vi "rqcBob Mod Level Test - 2 SPD (Low Level Example).vi"() -> ()   [LabVIEW 2018]
uses:
  FPGA/rqcBob/Custom Controls/Pulse Train/rqcBob Pulse Train Config.ctl
  FPGA/rqcBob/Custom Controls/Pulse Train/rqcBob Pulse Train.Generation Mode.ctl
  FPGA/rqcBob/Custom Controls/Pulse Train/rqcBob Pulse Train.First Pulse Delay Mode.ctl
  FPGA/rqcBob/Custom Controls/rqcBob Modulator Config.ctl
  FPGA/rqcBob/Custom Controls/rqcBob Window Config.ctl
  Shared/Shared FPGA Lib/Shared Logic/Custom Controls/rqc Random Generator.parameters.ctl
  Shared/Shared FPGA Lib/Shared Logic/Custom Controls/rqc Random Generator.value type.ctl
  FPGA/rqcBob/Custom Controls/rqcBob Trigger Type.ctl
  <vilib>/Analysis/1siggen.llb/Ramp Pattern by Delta.vi
  <vilib>/FPGAPlugInAG/PCI-7811R/niLvFpga_Open_PCI-7811R.vi
  <vilib>/rvi/interface/common/dynamic/niFpgaDynamicAddResources.vi
  Low Level API/Configuration/Photon Detector/Detection FIFOs config/rqcBob Configure PD Detect FIFO (2PD).vi
  Low Level API/Read/Read PD Detection FIFO/rqcBob Read PD Detection FIFO (1PD PD1).vi
  Low Level API/Read/Read PD Detection FIFO/rqcBob Read PD Detection FIFO (1PD PD2).vi
  <vilib>/FPGAPlugInAG/Dynamic/niLvFpga_Close_Dynamic.vi
  <vilib>/rvi/interface/nirviOpenFPGA/nirviOpenFPGA.xnode
  FPGA Bitfiles/rqcBob (FPGA) 7811 v 4.0.0.lvbitx
  <vilib>/rvi/interface/nirviCloseFPGA/nirviCloseFPGA.xnode
  <vilib>/Analysis/NI_AALBase.lvlib
panel:
  out "Num of Detections (2-nd PD) vs DAC Level":cluster{u16[], "appended array":dbl[]}(graph)={[0, 8, 16, 24, 32, 40, 48, 56, 64, 72, 80, 88, 96, 104, 112, 120, 128, 136, 144, 152, 160, 168, 176, 184, 192, 200, 208, 216, 224, 232, 240, 248, 256, 264, 272, 280, 288, 296, 304, 312, 320, 328, 336, 344, 352, 360, 368, 376, 384, 392, 400, 408, 416, 424, 432, 440, 448, 456, 464, 472, 480, 488, 496, 504, 512], "appended array"=[0.0, 0.0, 0.0, 0.0, 0.0, 0.0, 0.0, 0.0, 0.0, 0.0, 0.0, 0.0, 0.0, 0.0, 0.0, 0.0, 0.0, 0.0, 0.0, 0.0, 0.0, 0.0, 0.0, 0.0, 0.0, 0.0, 0.0, 0.0, 0.0, 0.0, 0.0, 0.0, 0.0, 0.0, 0.0, 0.0, 0.0, 0.0, 0.0, 0.0, 0.0, 0.0, 0.0, 0.0, 0.0, 0.0, 0.0, 0.0, 0.0, 0.0, 0.0, 0.0, 0.0, 0.0, 0.0, 0.0, 0.0, 0.0, 0.0, 0.0, 0.0, 0.0, 0.0, 0.0, 0.0]}
  in  "modulator.clock delay":fxp<+,4,4> caption="PM Clock Delay (0-7) (in units of 40ns)"
  out "Progress":dbl(slide)=100.0 scale=0.0..100.0
  out "Num of Detections (1-st PD) vs DAC Level":cluster{u16[], "appended array":dbl[]}(graph)={[0, 8, 16, 24, 32, 40, 48, 56, 64, 72, 80, 88, 96, 104, 112, 120, 128, 136, 144, 152, 160, 168, 176, 184, 192, 200, 208, 216, 224, 232, 240, 248, 256, 264, 272, 280, 288, 296, 304, 312, 320, 328, 336, 344, 352, 360, 368, 376, 384, 392, 400, 408, 416, 424, 432, 440, 448, 456, 464, 472, 480, 488, 496, 504, 512], "appended array"=[0.0, 0.0, 0.0, 0.0, 0.0, 0.0, 0.0, 0.0, 0.0, 0.0, 0.0, 0.0, 0.0, 0.0, 0.0, 0.0, 0.0, 0.0, 0.0, 0.0, 0.0, 0.0, 0.0, 0.0, 0.0, 0.0, 0.0, 0.0, 0.0, 0.0, 0.0, 0.0, 0.0, 0.0, 0.0, 0.0, 0.0, 0.0, 0.0, 0.0, 0.0, 0.0, 0.0, 0.0, 0.0, 0.0, 0.0, 0.0, 0.0, 0.0, 0.0, 0.0, 0.0, 0.0, 0.0, 0.0, 0.0, 0.0, 0.0, 0.0, 0.0, 0.0, 0.0, 0.0, 0.0]}
  in  "stop":bool
  in  "DAC increment":u16=8
  in  "DAC Level max":u16=512
  in  "DAC Level min":u16
  in  "rndGen.parameters":T1={"value type"=enum."constant", "constant"=512, "num of levels"=0, "levels values"=[0, 0, 0, 0]} caption="Phase modulation value" {"num of levels" min=4 max=4 step=1}
  in  "window.config":T3 caption="Registration of detector clicks"
  in  "modulator.config":T4 caption="Phase modulation"
  in  "train.configuration":T5={"period"=0, "num of pulses"=0, "mode"=enum."train sequence.single", "num of trains"=0, "first pulse delay mode"=enum."every train", "first pulse delay"=55} caption="Pulsed laser configuration"
  out "Done":bool=TRUE
  # "PM Level Settings"
  # "Bob configuration"
  # "Advanced parameters"
  # "Constant"
  # "Random"
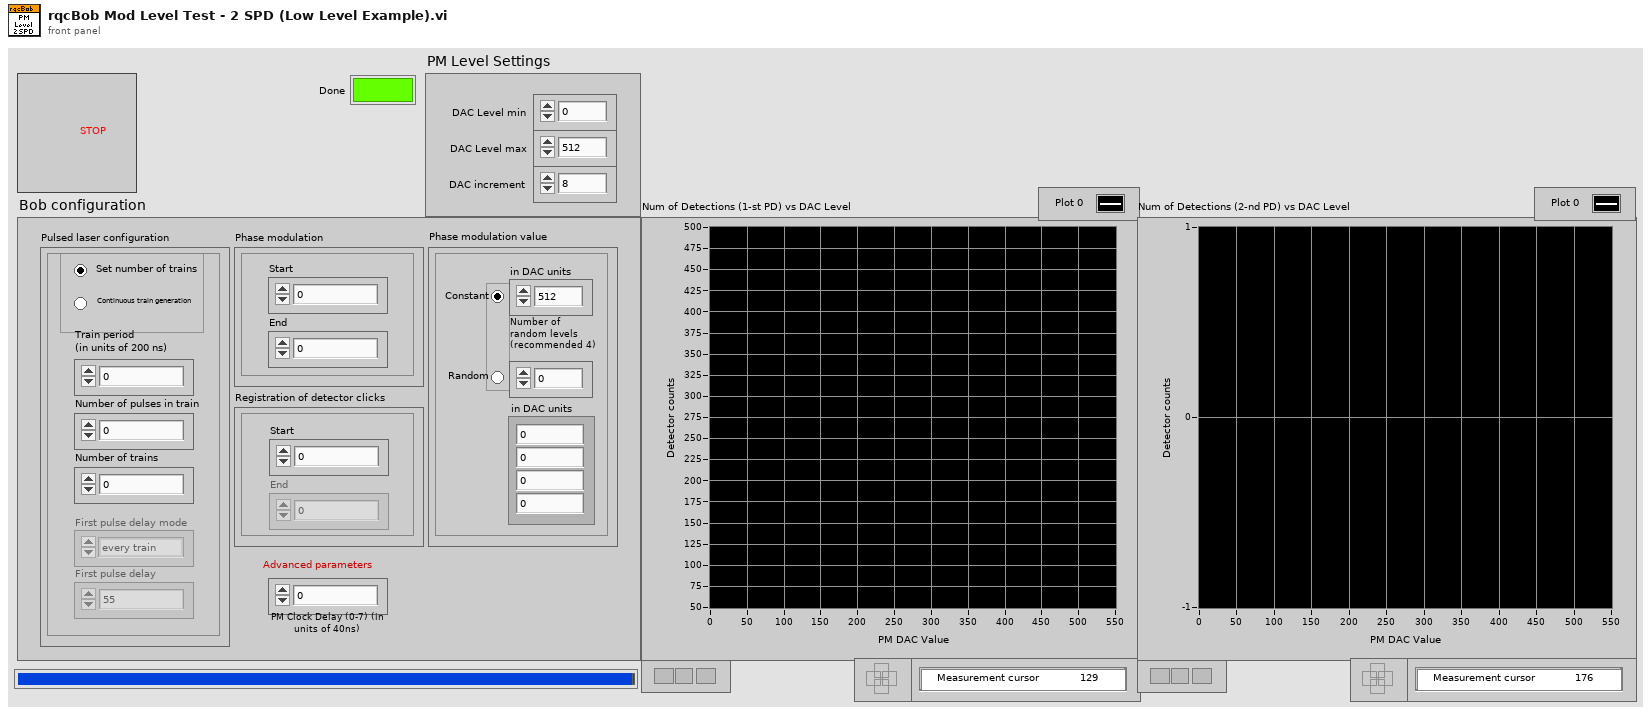
[diagram p1: front panel]
types:
  T1 = typedef "rqc Random Generator.parameters.ctl" = cluster{"value type":T2, "constant":u16, "num of levels":u16, "levels values":u16[]}
  T2 = typedef "rqc Random Generator.value type.ctl" = enum32{"random value", "constant"}
  T3 = typedef "rqcBob Window Config.ctl" = cluster{"window.open":u16, "window.close":u16}
  T4 = typedef "rqcBob Modulator Config.ctl" = cluster{"modulator.start":u16, "modulator.stop":u16}
  T5 = typedef "rqcBob Pulse Train Config.ctl" = cluster{"period":u16, "num of pulses":u16, "mode":T6, "num of trains":u16, "first pulse delay mode":T7, "first pulse delay":u16}
  T6 = typedef "rqcBob Pulse Train.Generation Mode.ctl" = enum32{"single train", "train sequence.single", "train sequence.wait for trigger", "continuous"}
  T7 = typedef "rqcBob Pulse Train.First Pulse Delay Mode.ctl" = enum8{"none", "every train", "first train"}
  T8 = typedef "rqcBob Trigger Type.ctl" = enum16{"software", "immediate", "DIO"}
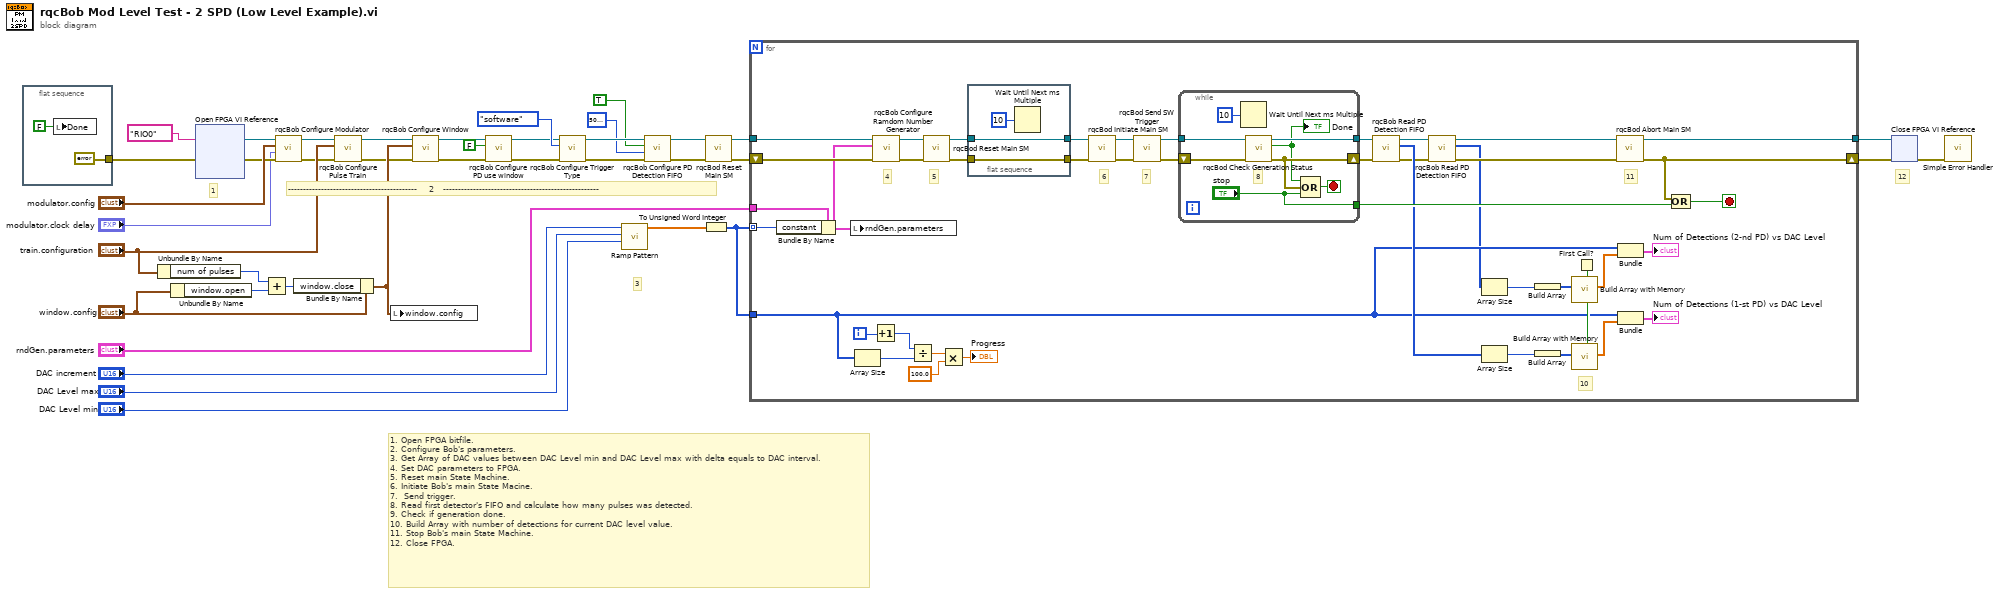
[diagram p0: block diagram]
diagram:
  # "12"
  # "3"
  # "1. Open FPGA bitfile.\n2. Configure Bob's parameters.\n3. Get Array of DAC values between DAC Level min and DAC Level max with delta equals to DAC interval.\n4. Set DAC parameters to FPGA.\n5. Reset main State Machine.\n6. Initiate Bob's main State Macine.\n7.  Send trigger.\n8. Read first detector's FIFO and calculate how many pulses was detected.\n9. Check if generation done.\n10. Build Array with number of detections for current DAC level value.\n11. Stop Bob's main State Machine.\n12. Close FPGA."
  # "1"
  # "-------------------------------------------    2   ----------------------------------------------------"
  n1 = flat-sequence {
    tunnel: [errorcluster {"status"=FALSE, "code"=0, "source"=""} ("error in")] -> w36
    frame #0 {
      n2 = local write "Done"(FALSE ("Done")) -> ()
    }
  }
  n3 = Unbundle By Name("train.configuration") -> ("num of pulses"=w34:u16)
  n4 = Unbundle By Name("window.config") -> ("window.open"=w33:u16)
  n5 = xnode "Open FPGA VI Reference"("error in"=w36, "resource name"=tag "RIO0") -> ("FPGA VI Reference Out"=w11:refnum<k20>, "error out"=w10:errorcluster)
  n6 = Add(x=w34, y=w33) -> (x+y=w31:u16)
  n7 = call "rqcBob Configure Modulator.vi"("error in"=w10, "modulator.clock delay"="modulator.clock delay", "modulator.config"="modulator.config", "FPGA reference in"=w11) -> ("error out"=w24:errorcluster, "FPGA reference out"=w25:refnum<k20>)  [unwired: 6 in]
  n8 = Bundle By Name(cluster="window.config", "window.close"=w31) -> (w30:T3)
  n9 = call "rqcBob Configure Pulse Train.vi"("error in"=w24, "train.configuration"="train.configuration", "FPGA reference in"=w25) -> ("error out"=w26:errorcluster, "FPGA reference out"=w27:refnum<k20>)  [unwired: 6 in, 1 out]
  n10 = local write "window.config"(w30) -> ()
  n11 = call "rqcBob Configure Window.vi"("error in"=w26, "window.config"=w30, "FPGA reference in"=w27) -> ("error out"=w28:errorcluster, "FPGA reference out"=w29:refnum<k20>)  [unwired: 7 in]
  n12 = call "rqcBob Configure PD use window.vi"("error in"=w28, "PD.use window"=FALSE ("SPD.use detector window"), "FPGA reference in"=w29) -> ("error out"=w1:errorcluster, "FPGA reference out"=w2:refnum<k20>)  [unwired: 7 in]
  n13 = call "rqcBob Configure Trigger Type.vi"("error in"=w1, "rqcBob Trigger Type"=rqcBob_Trigger_Type."software", "FPGA reference in"=w2) -> ("error out"=w6:errorcluster, "FPGA reference out"=w8:refnum<k20>)  [unwired: 7 in]
  n14 = call-poly <vilib>:"Ramp Pattern.vi"("start"="DAC Level min", "end"="DAC Level max", "delta"="DAC increment") -> ("Ramp Pattern"=w20:dbl[])  [unwired: 6 in, 2 out]
  n15 = call-poly "rqcBob Configure PD Detection FIFO.vi"("error in"=w6, "PD.detect fifo depth"=u32 5000000 ("SPD.detect fifo depth"), "PD.detect fifo write enable"=TRUE ("SPD.detect fifo write enable"), "FPGA reference in"=w8) -> ("error out"=w3:errorcluster, "FPGA reference out"=w7:refnum<k20>)  [unwired: 6 in]
  n16 = To Unsigned Word Integer(number=w20) -> (unsigned 16bit integer=w19:u16[])
  n17 = call "rqcBod Reset Main SM.vi"("error in"=w3, "FPGA reference in"=w7) -> ("error out"=w13:errorcluster, "FPGA reference out"=w14:refnum<k20>)  [unwired: 8 in]
  n18 = for {
    tunnel: w14 -> [w82]
    tunnel: w19 -> [w56] mode=indexing
    tunnel: "rndGen.parameters" -> [w80]
    tunnel: [w77] -> w18
    shift-right: [w75] -> w17
    shift-left: w13 -> [w81]
    tunnel: w19 -> [w43]
    i -> [w65]
    stop <- w73 stop-if-true
    # "5"
    # "11"
    # "10"
    # "7"
    # "6"
    # "4"
    n19 = Bundle By Name(cluster=w80, "constant"=w56) -> (w74:T1)
    n20 = local write "rndGen.parameters"(w74) -> ()
    n21 = Array Size(array=w43) -> (size(s)=w72:i32)
    n22 = Increment(x=w65) -> (x+1=w71:i32)
    n23 = call "rqcBob Configure Ramdom Number Generator.vi"("error in"=w81, "rqcBob rndGen.parameters"=w74, "FPGA reference in"=w82) -> ("error out"=w61:errorcluster, "FPGA reference out"=w62:refnum<k20>)  [unwired: 7 in]
    n24 = Divide(x=w71, y=w72) -> (x/y=w70:dbl)
    n25 = call "rqcBod Reset Main SM.vi"("error in"=w61, "FPGA reference in"=w62) -> ("error out"=w57:errorcluster, "FPGA reference out"=w58:refnum<k20>)  [unwired: 8 in]
    n26 = Multiply(x=w70, y=100.0) -> (x*y=→"Progress":dbl)
    n27 = flat-sequence {
      tunnel: [w87] -> w60
      tunnel: w58 -> [w87]
      tunnel: [w86] -> w59
      tunnel: w57 -> [w86]
      frame #0 {
        n28 = Wait Until Next ms Multiple(millisecond multiple=u32 10) -> ()  [unwired: 1 out]
      }
    }
    n29 = call "rqcBod Initiate Main SM.vi"("error in"=w59, "FPGA reference in"=w60) -> ("error out"=w83:errorcluster, "FPGA reference out"=w84:refnum<k20>)  [unwired: 8 in]
    n30 = call "rqcBod Send SW Trigger.vi"("error in"=w83, "FPGA reference in"=w84) -> ("error out"=w78:errorcluster, "FPGA reference out"=w79:refnum<k20>)  [unwired: 8 in]
    n31 = while {
      tunnel: w79 -> [w90]
      shift-right: [w95] -> w54
      shift-left: w78 -> [w91]
      tunnel: [w89] -> w55
      tunnel: ["stop"] -> w76
      stop <- w94 stop-if-true
      # "8"
      n32 = Wait Until Next ms Multiple(millisecond multiple=u32 10) -> ()  [unwired: 1 out]
      n33 = call "rqcBod Check Generation Status.vi"("error in"=w91, "FPGA reference in"=w90) -> ("error out"=w95:errorcluster, "generation.done"=w88:bool, "FPGA reference out"=w89:refnum<k20>)  [unwired: 7 in]
      "Done" <- w88
      n34 = Compound Arithmetic op=OR(w88, w95, "stop") -> (w94:bool)
    }
    n35 = call-poly "rqcBob Read PD Detection FIFO.vi"("error in"=w54, "FPGA reference in"=w55) -> ("error out"=w51:errorcluster, "Data"=w53:u32[], "FPGA reference out"=w52:refnum<k20>)  [unwired: 6 in, 1 out]
    n36 = call-poly "rqcBob Read PD Detection FIFO.vi"("error in"=w51, "FPGA reference in"=w52) -> ("error out"=w50:errorcluster, "Data"=w42:u32[], "FPGA reference out"=w49:refnum<k20>)  [unwired: 6 in, 1 out]
    n37 = Array Size(array=w42) -> (size(s)=w48:i32)
    n38 = Array Size(array=w53) -> (size(s)=w63:i32)
    n39 = Build Array(w48) -> (w46:i32[])
    n40 = Build Array(w63) -> (w66:i32[])
    n41 = First Call?() -> (First Call?: T/F=w44:bool)
    n42 = call "Build Array with Memory.vi"("reset"=w44, "new array"=w46) -> ("appended array"=w45:dbl[])  [unwired: 9 in]
    n43 = call "Build Array with Memory.vi"("reset"=w44, "new array"=w66) -> ("appended array"=w67:dbl[])  [unwired: 9 in]
    n44 = call "rqcBod Abort Main SM.vi"("error in"=w50, "FPGA reference in"=w49) -> ("error out"=w75:errorcluster, "FPGA reference out"=w77:refnum<k20>)  [unwired: 8 in]
    n45 = Bundle(w43, "appended array"=w45) -> (→"Num of Detections (2-nd PD) vs DAC Level":cluster{u16[], "appended array":dbl[]})  [unwired: 1 in]
    n46 = Bundle(w43, "appended array"=w67) -> (→"Num of Detections (1-st PD) vs DAC Level":cluster{u16[], "appended array":dbl[]})  [unwired: 1 in]
    n47 = Compound Arithmetic op=OR(w75, w76) -> (w73:bool)
  }
  n48 = xnode "Close FPGA VI Reference"("FPGA VI Reference In"=w18, "error in"=w17) -> ("error out"=w16:errorcluster)
  n49 = call <vilib>:"Simple Error Handler.vi"("error in (no error)"=w16) -> ()  [unwired: 4 in, 5 out]
